vi "NewTurretControlTest.vi"() -> ()   [LabVIEW 2020]
panel:
  out "goal":dbl
  in  "TurretTarget":dbl
  in  "TurretAngle":dbl
  in  "RobotHeading":dbl
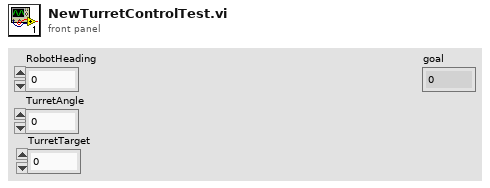
[diagram p1: front panel]
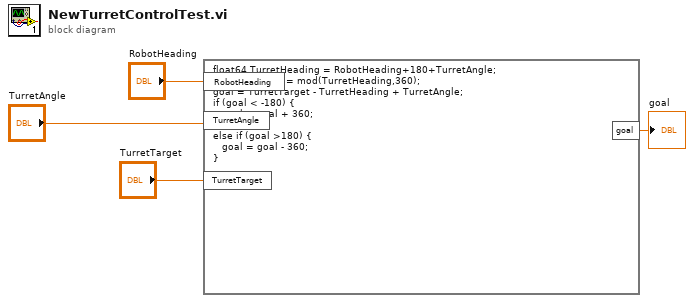
[diagram p0: block diagram]
diagram:
  n1 = formula code="float64 TurretHeading = RobotHeading+180+TurretAngle;\nTurretHeading = mod(TurretHeading,360);\ngoal = TurretTarget - TurretHeading + TurretAngle;\nif (goal < -180) {\n   goal = goal + 360;\n} \nelse if (goal >180) {\n   goal = goal - 360;\n}"("TurretAngle"="TurretAngle", "RobotHeading"="RobotHeading", "TurretTarget"="TurretTarget") -> ("goal"=→"goal":dbl)
